vi "SetBoundsBySocket.vi"(8 "Error In":errorcluster, 9 "Test Name":string, 10 "Number of Sockets":i32, 11 "Test Socket":i32) -> (0 "Error Out":errorcluster)   [LabVIEW 2013]
uses:
  <vilib>/Utility/miscctls.llb/LVRectTypeDef.ctl
panel:
  out "Display:Primary Workspace":T1
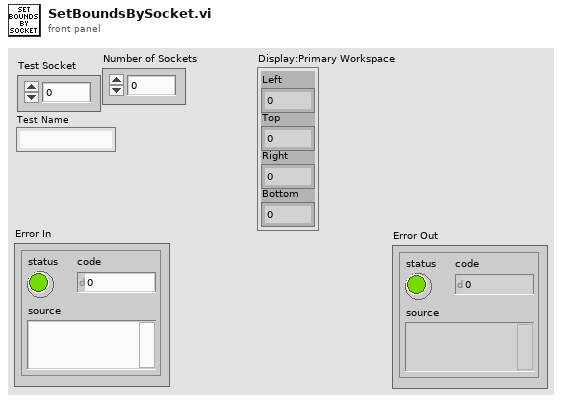
[diagram p1: front panel]
types:
  T1 = typedef "LVRectTypeDef.ctl" = cluster{"Left":i16, "Top":i16, "Right":i16, "Bottom":i16}
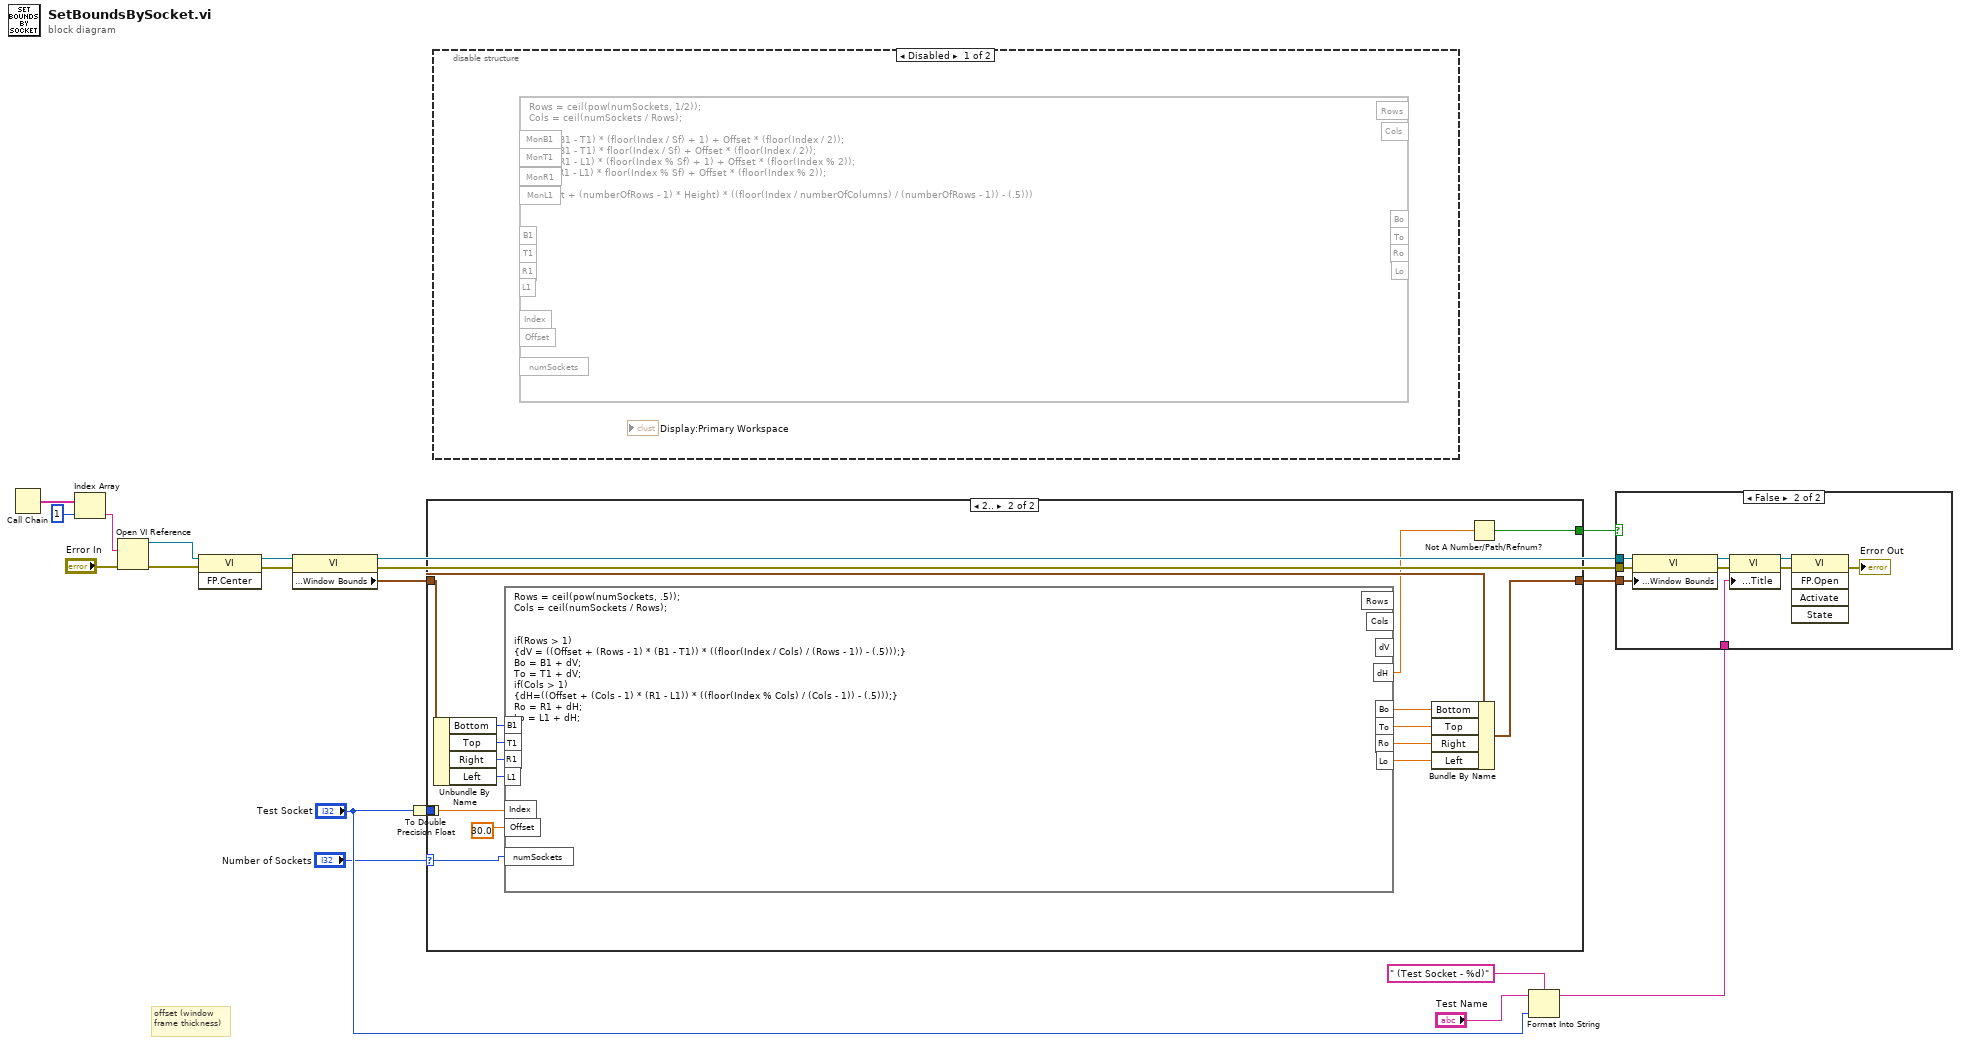
[diagram p0: block diagram]
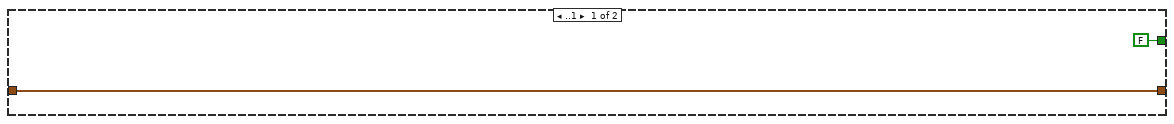
[diagram p2: hidden frame]
diagram:
  # "offset (window frame thickness)"
  n1 = Call Chain() -> (call chain=w18:string[])
  n2 = Index Array(array=w18, index=1) -> (element=w16:string)
  n3 = Open VI Reference(vi path=w16, error in (no error)="Error In") -> (vi reference=w6:refnum<vi>, error out=w5:errorcluster)  [unwired: 4 in]
  n4 = invoke class="VI" method="FP.Center"(reference=w6, error in=w5) -> (reference out=w7:refnum<vi>, error out=w4:errorcluster)  [unwired: 1 in, 1 out]
  n5 = property class="VI"(reference=w7, error in=w4) -> (reference out=w15:refnum<vi>, error out=w10:errorcluster, "Front Panel Window:Window Bounds"=w8:T1)
  n6 = case shown="2.." "Number of Sockets" {
    selector: "Number of Sockets" -> [_ w21]
    tunnel: [w19 w31] -> w9
    tunnel: w8 -> [w19 w30]
    tunnel: "Test Socket" -> [_ w25]
    tunnel: [FALSE w22] -> w2
    frame ..1 {
    }
    frame 2.. {
      n7 = To Double Precision Float(number=w25) -> (double precision float=w24:dbl)
      n8 = Unbundle By Name(w30) -> ("Bottom"=w35:i16, "Top"=w34:i16, "Right"=w33:i16, "Left"=w32:i16)
      n9 = formula code="Rows = ceil(pow(numSockets, .5));\nCols = ceil(numSockets / Rows);\n\n\nif(Rows > 1)\n{dV = ((Offset + (Rows - 1) * (B1 - T1)) * ((floor(Index / Cols) / (Rows - 1)) - (.5)));}\nBo = B1 + dV;\nTo = T1 + dV;\nif(Cols > 1)\n{dH=((Offset + (Cols - 1) * (R1 - L1)) * ((floor(Index % Cols) / (Cols - 1)) - (.5)));}\nRo = R1 + dH;\nLo = L1 + dH;"("B1"=w35, "T1"=w34, "R1"=w33, "L1"=w32, "Index"=w24, "Offset"=30.0, "numSockets"=w21) -> ("Bo"=w29:dbl, "To"=w28:dbl, "Ro"=w27:dbl, "Lo"=w26:dbl, "dH"=w23:dbl)  [unwired: 3 out]
      n10 = Bundle By Name(cluster=w30, "Bottom"=w29, "Top"=w28, "Right"=w27, "Left"=w26) -> (w31:T1)
      n11 = Not A Number/Path/Refnum?(number/path/refnum=w23) -> (NaN/Path/Refnum?=w22:bool)
    }
  }
  n12 = disable-structure shown="Disabled" {
    frame Disabled {
      n13 = formula code="Rows = ceil(pow(numSockets, 1/2));\nCols = ceil(numSockets / Rows);\n\nBo = (B1 - T1) * (floor(Index / Sf) + 1) + Offset * (floor(Index / 2));\nTo = (B1 - T1) * floor(Index / Sf) + Offset * (floor(Index / 2));\nRo = (R1 - L1) * (floor(Index % Sf) + 1) + Offset * (floor(Index % 2));\nLo = (R1 - L1) * floor(Index % Sf) + Offset * (floor(Index % 2));\n\n((Offset + (numberOfRows - 1) * Height) * ((floor(Index / numberOfColumns) / (numberOfRows - 1)) - (.5)))"() -> ()  [unwired: 11 in, 6 out]
    }
    frame Enabled {
    }
  }
  n14 = Format Into String(format string=" (Test Socket - %d)", initial string="Test Name", "Test Socket") -> (resulting string=w12:string)  [unwired: 1 in, 1 out]
  n15 = case shown="False" w2 {
    tunnel: w15 -> [_ w45]
    tunnel: w12 -> [_ w43]
    tunnel: w10 -> [_ w42]
    tunnel: w9 -> [_ w37]
    frame True {
    }
    frame False {
      n16 = property class="VI"(reference=w45, error in=w42, "Front Panel Window:Window Bounds"=w37) -> (reference out=w44:refnum<vi>, error out=w41:errorcluster)
      n17 = property class="VI"(reference=w44, error in=w41, "Front Panel.Title"=w43) -> (reference out=w38:refnum<vi>, error out=w40:errorcluster)
      n18 = invoke class="VI" method="FP.Open"(reference=w38, error in=w40) -> (error out=→"Error Out":errorcluster)  [unwired: 3 in, 4 out]
    }
  }
